vi "Write Cluster to PGSQL.vi"(8 "error in (no error)":errorcluster, 9 "Variant":variant, 10 "Process name":string, 11 "Logger in":refnum<class "Logger.PGSQL.lvclass">) -> (0 "error out":errorcluster, 3 "Logger out":refnum<class "Logger.PGSQL.lvclass">)   [LabVIEW 2016, in "Logger.PGSQL.lvclass"]
uses:
  Logger.PGSQL.lvclass
  <vilib>/Utility/Data Type/NI_Data Type.lvlib
  <resource>/objmgr/ni.var.rc
  <vilib>/JKI/JKI SMO/URI Parsing/URI.lvlib
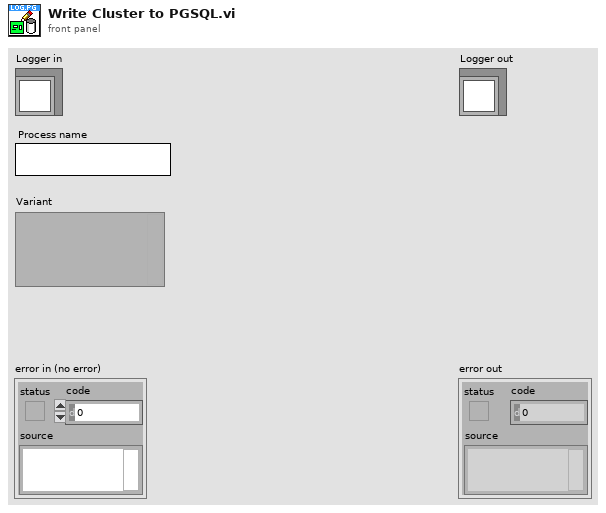
[diagram p1: front panel]
types:
  T1 = typedef "NI_Data Type.lvlib/Data Type.ctl" = enum8{"Invalid Type", "Void", "I8", "I16", "I32", "I64", "U8", "U16", "U32", "U64", "Single Float", "Double Float", "Extended Float", "Single Complex", "Double Complex", "Extended Complex", "Enum U8", "Enum U16", "Enum U32", "Enum U64", "Single Float With Unit", "Double Float With Unit", "Extended Float With Unit", "Single Complex with Unit", "Double Complex with Unit", "Extended Complex with Unit", "Boolean", "String", "Path", "Picture", "Tag", "Array", "Cluster", "Variant", "LV Variant", "Waveform", "Timestamp", "Digital Waveform", "Digital Data", "ExpressData", "Refnum", "External Data", "VI", "Poly VI", "LabVIEW Class Instance", "Fixed Point"}
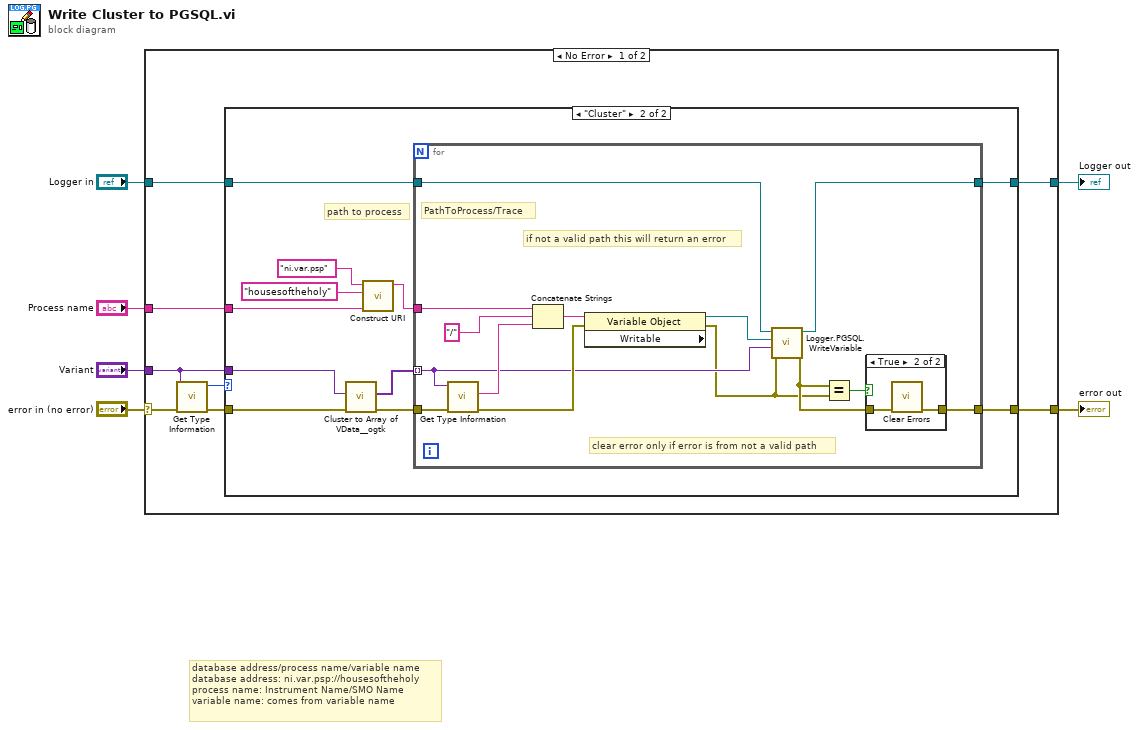
[diagram p0: block diagram]
diagram:
  # "database address/process name/variable name\ndatabase address: ni.var.psp://housesoftheholy\nprocess name: Instrument Name/SMO Name\nvariable name: comes from variable name"
  n1 = case shown="No Error" "error in (no error)" {
    selector: "error in (no error)" -> [w12 w46]
    tunnel: [w9 w46] -> w5
    tunnel: [w8 w45] -> w3
    tunnel: "Logger in" -> [w10 w45]
    tunnel: "Variant" -> [w7 _]
    tunnel: "Process name" -> [w11 _]
    frame No Error {
      n2 = call <vilib>:"Get Type Information.vi"("error in (no error)"=w12, "Variant"=w7) -> ("error out"=w13:errorcluster, "Type"=w14:T1)  [unwired: 5 in, 3 out]
      n3 = case shown="\"Cluster\"" w14 {
        tunnel: w11 -> [_ w17]
        tunnel: [w16 w26] -> w9
        tunnel: w7 -> [_ w25]
        tunnel: w13 -> [w16 w23]
        tunnel: [w15 w22] -> w8
        tunnel: w10 -> [w15 w21]
        frame Default {
        }
        frame "Cluster" {
          # "path to process"
          n4 = call <userlib>:"Cluster to Array of VData__ogtk.vi"("error in (no error)"=w23, "Cluster"=w25) -> ("error out"=w27:errorcluster, "Array of VData"=w24:variant[])  [unwired: 8 in]
          n5 = call <vilib>:"Construct URI.vi"("path"=w17, "address"="housesoftheholy", "protocol"="ni.var.psp") -> ("URI"=w18:string)  [unwired: 8 in]
          n6 = for {
            tunnel: w24 -> [w34] mode=indexing
            tunnel: w27 -> [w41]
            tunnel: w18 -> [w39]
            tunnel: [w32] -> w26
            tunnel: w21 -> [w33]
            tunnel: [w28] -> w22
            # "clear error only if error is from not a valid path"
            # "PathToProcess/Trace"
            # "if not a valid path this will return an error"
            n7 = call <vilib>:"Get Type Information.vi"("error in (no error)"=w41, "Variant"=w34) -> ("error out"=w36:errorcluster, "Name"=w40:string)  [unwired: 5 in, 3 out]
            n8 = Concatenate Strings(w39, "/" ("string"), w40) -> (w37:string)
            n9 = property class="Variable Object" props=["Writable"](reference=w37, error in=w36) -> (reference out=w35:refnum<k21>, error out=w30:errorcluster)  [unwired: 1 out]
            n10 = call "Logger.PGSQL.WriteVariable.vi"("error in (no error)"=w30, "Data"=w34, "Address"=w35, "Logger"=w33) -> ("error out"=w31:errorcluster, "Logger out"=w28:refnum<class "Logger.PGSQL.lvclass">)  [unwired: 6 in]
            n11 = Equal?(x=w31, y=w30) -> (x = y?=w29:bool)
            n12 = case shown="True" w29 {
              tunnel: [w42 w44] -> w32
              tunnel: w31 -> [w42 w43]
              frame False {
              }
              frame True {
                n13 = call <vilib>:"Clear Errors.vi"("error in (no error)"=w43) -> ("error out"=w44:errorcluster)  [unwired: 5 in, 1 out]
              }
            }
          }
        }
      }
    }
    frame Error {
    }
  }
  "error out" <- w5
  "Logger out" <- w3
